vi "Sequence.CreateConditions.vi"(6 "Skip":T1, 8 "error in (no error)":errorcluster, 9 "Condition":T2, 10 "Iteration":string, 11 "Task":refnum<k24>) -> (0 "error out":errorcluster, 3 "Tasks":refnum<k24>[](array[refnum]))   [LabVIEW 2015, in "Single Station Execution.lvlib"]
uses:
  Single Station Execution.lvlib
  NationalInstruments.VeriStand.RealTimeSequenceDefinitionApi
  Types/Compiled.StepCondition.ctl
  Types/Conditions.OperationTypes.ctl
  Types/Channel.Properties.ctl
  Main.Constants.vi
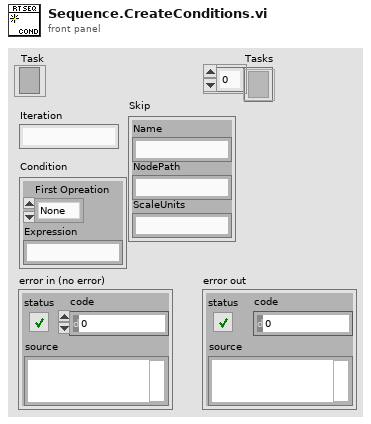
[diagram p1: front panel]
types:
  T1 = typedef "Single Station Execution.lvlib/Channel.Properties.ctl" = cluster{"Name":string, "NodePath":string, "ScaleUnits":string}
  T2 = typedef "Single Station Execution.lvlib/Compiled.StepCondition.ctl" = cluster{"First Opreation":T3, "Expression":string}
  T3 = typedef "Single Station Execution.lvlib/Conditions.OperationTypes.ctl" = enum8{"None", "&&", "||"}
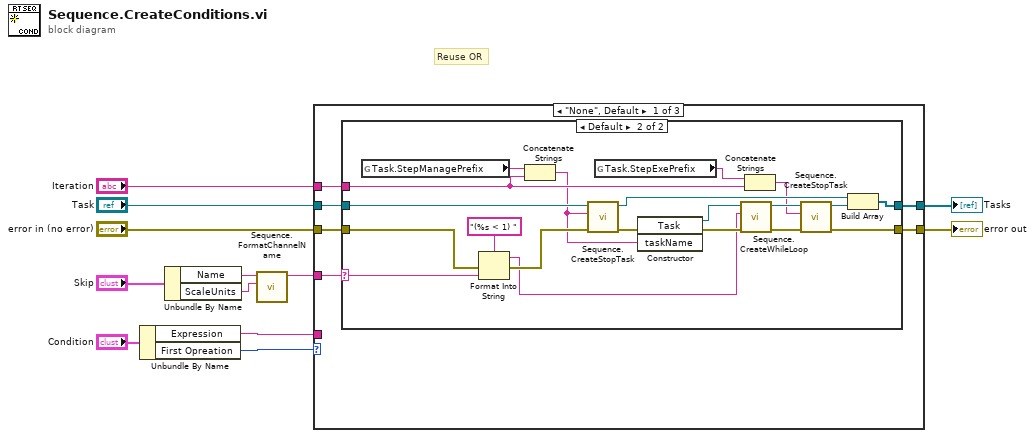
[diagram p0: block diagram]
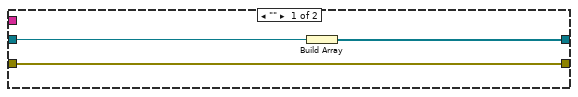
[diagram p2: hidden frame]
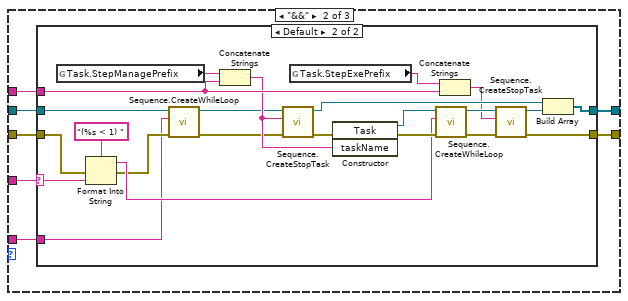
[diagram p3: hidden frame]
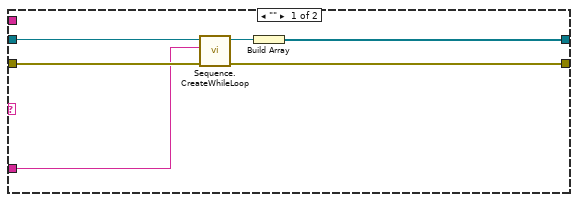
[diagram p4: hidden frame]
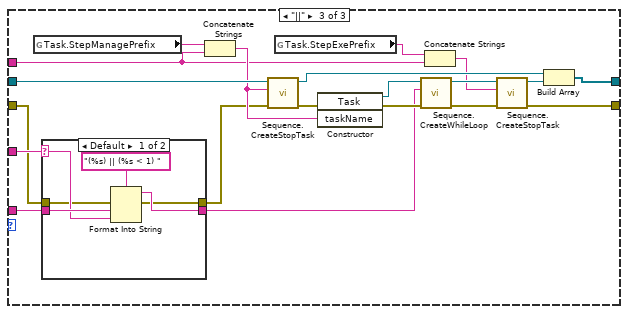
[diagram p5: hidden frame]
diagram:
  # "Reuse OR"
  n1 = Unbundle By Name("Condition") -> ("Expression"=w9:string, "First Opreation"=w8:T3)
  n2 = Unbundle By Name("Skip") -> ("Name"=w3:string, "ScaleUnits"=w2:string)
  n3 = call "Sequence.FormatChannelName.vi"("ScaleUnits"=w2, "Name"=w3) -> ("ChannelName"=w1:string)  [unwired: 9 in]
  n4 = case shown="\"None\", Default" w8 {
    tunnel: [w15 w43 w87] -> w11
    tunnel: "error in (no error)" -> [w18 w46 w79]
    tunnel: "Task" -> [w17 w47 w92]
    tunnel: "Iteration" -> [w16 w48 w85]
    tunnel: w9 -> [_ w44 w81]
    tunnel: [w14 w42 w88] -> w10
    tunnel: w1 -> [w13 w45 w82]
    frame "None", Default {
      n5 = case shown="Default" w13 {
        selector: w13 -> [_ w22]
        tunnel: w18 -> [w21 w29]
        tunnel: w17 -> [w20 w28]
        tunnel: w16 -> [_ w27]
        tunnel: [w21 w24] -> w15
        tunnel: [w19 w23] -> w14
        frame "" {
          n6 = Build Array(w20) -> (w19:refnum<k24>[])
        }
        frame Default {
          n7 = global read "Main.Constants.vi" "Task.StepManagePrefix"() -> (w32:string)
          n8 = Format Into String(format string="(%s < 1) ", error in=w29, w22) -> (resulting string=w25:string, error out=w30:errorcluster)  [unwired: 1 in]
          n9 = Concatenate Strings(w32, w27) -> (w26:string)
          n10 = call "Sequence.CreateStopTask.vi"("error in (no error)"=w30, "Task Name"=w26, "Task Ref"=w28) -> ("error out"=w35:errorcluster, ".NET Refnum out"=w36:refnum<k24>)  [unwired: 7 in]
          n11 = global read "Main.Constants.vi" "Task.StepExePrefix"() -> (w34:string)
          n12 = constructor class="Task"(error in=w35, "taskName"=w26) -> (reference out=w41:refnum<k24>, error out=w40:errorcluster)  [unwired: 2 in, 2 out]
          n13 = call "Sequence.CreateWhileLoop.vi"("error in (no error)"=w40, "Expression"=w25, "Task Ref"=w41) -> ("error out"=w37:errorcluster, "Task Ref out"=w39:refnum<k24>)  [unwired: 7 in]
          n14 = Concatenate Strings(w34, w27) -> (w33:string)
          n15 = call "Sequence.CreateStopTask.vi"("error in (no error)"=w37, "Task Name"=w33, "Task Ref"=w39) -> ("error out"=w24:errorcluster, ".NET Refnum out"=w38:refnum<k24>)  [unwired: 7 in]
          n16 = Build Array(w36, w38) -> (w23:refnum<k24>[])
        }
      }
    }
    frame "&&" {
      n17 = case shown="Default" w45 {
        selector: w45 -> [_ w60]
        tunnel: w46 -> [w51 w66]
        tunnel: w47 -> [w53 w58]
        tunnel: w48 -> [_ w65]
        tunnel: [w52 w62] -> w43
        tunnel: [w50 w61] -> w42
        tunnel: w44 -> [w49 w55]
        frame "" {
          n18 = call "Sequence.CreateWhileLoop.vi"("error in (no error)"=w51, "Expression"=w49, "Task Ref"=w53) -> ("error out"=w52:errorcluster, "Task Ref out"=w54:refnum<k24>)  [unwired: 7 in]
          n19 = Build Array(w54) -> (w50:refnum<k24>[])
        }
        frame Default {
          n20 = global read "Main.Constants.vi" "Task.StepManagePrefix"() -> (w68:string)
          n21 = Format Into String(format string="(%s < 1) ", error in=w66, w60) -> (resulting string=w63:string, error out=w57:errorcluster)  [unwired: 1 in]
          n22 = call "Sequence.CreateWhileLoop.vi"("error in (no error)"=w57, "Expression"=w55, "Task Ref"=w58) -> ("error out"=w56:errorcluster, "Task Ref out"=w59:refnum<k24>)  [unwired: 7 in]
          n23 = Concatenate Strings(w68, w65) -> (w64:string)
          n24 = call "Sequence.CreateStopTask.vi"("error in (no error)"=w56, "Task Name"=w64, "Task Ref"=w59) -> ("error out"=w71:errorcluster, ".NET Refnum out"=w72:refnum<k24>)  [unwired: 7 in]
          n25 = global read "Main.Constants.vi" "Task.StepExePrefix"() -> (w70:string)
          n26 = constructor class="Task"(error in=w71, "taskName"=w64) -> (reference out=w77:refnum<k24>, error out=w76:errorcluster)  [unwired: 2 in, 2 out]
          n27 = call "Sequence.CreateWhileLoop.vi"("error in (no error)"=w76, "Expression"=w63, "Task Ref"=w77) -> ("error out"=w73:errorcluster, "Task Ref out"=w75:refnum<k24>)  [unwired: 7 in]
          n28 = Concatenate Strings(w70, w65) -> (w69:string)
          n29 = call "Sequence.CreateStopTask.vi"("error in (no error)"=w73, "Task Name"=w69, "Task Ref"=w75) -> ("error out"=w62:errorcluster, ".NET Refnum out"=w74:refnum<k24>)  [unwired: 7 in]
          n30 = Build Array(w72, w74) -> (w61:refnum<k24>[])
        }
      }
    }
    frame "||" {
      n31 = global read "Main.Constants.vi" "Task.StepManagePrefix"() -> (w83:string)
      n32 = case shown="Default" w82 {
        selector: w82 -> [w101 _]
        tunnel: w81 -> [w102 w105]
        tunnel: [w100 w105] -> w80
        tunnel: w79 -> [w99 w104]
        tunnel: [w98 w104] -> w78
        frame Default {
          n33 = Format Into String(format string="(%s) || (%s < 1) ", error in=w99, w102, w101) -> (resulting string=w100:string, error out=w98:errorcluster)  [unwired: 1 in]
        }
        frame "" {
        }
      }
      n34 = Concatenate Strings(w83, w85) -> (w89:string)
      n35 = call "Sequence.CreateStopTask.vi"("error in (no error)"=w78, "Task Name"=w89, "Task Ref"=w92) -> ("error out"=w90:errorcluster, ".NET Refnum out"=w91:refnum<k24>)  [unwired: 7 in]
      n36 = global read "Main.Constants.vi" "Task.StepExePrefix"() -> (w86:string)
      n37 = constructor class="Task"(error in=w90, "taskName"=w89) -> (reference out=w97:refnum<k24>, error out=w96:errorcluster)  [unwired: 2 in, 2 out]
      n38 = call "Sequence.CreateWhileLoop.vi"("error in (no error)"=w96, "Expression"=w80, "Task Ref"=w97) -> ("error out"=w93:errorcluster, "Task Ref out"=w95:refnum<k24>)  [unwired: 7 in]
      n39 = Concatenate Strings(w86, w85) -> (w84:string)
      n40 = call "Sequence.CreateStopTask.vi"("error in (no error)"=w93, "Task Name"=w84, "Task Ref"=w95) -> ("error out"=w87:errorcluster, ".NET Refnum out"=w94:refnum<k24>)  [unwired: 7 in]
      n41 = Build Array(w91, w94) -> (w88:refnum<k24>[])
    }
  }
  "error out" <- w11
  "Tasks" <- w10
